vi "Add Panel to SubPanel.vi"(10 "SubPanel Ref":i32, 11 "VI in":refnum<vi>) -> (0 "error out":errorcluster)   [LabVIEW 2015, in "Instrument.lvlib" / "Instrument.lvclass"]
uses:
  Instrument.lvclass
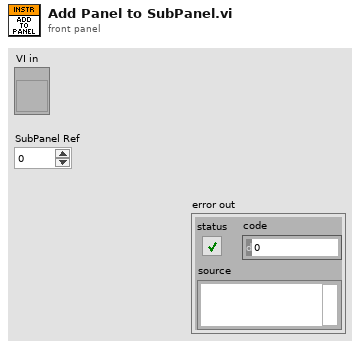
[diagram p1: front panel]
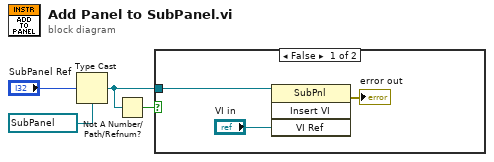
[diagram p0: block diagram]
diagram:
  n1 = Type Cast(type=refnum<vi> refnum ("Sub Panel"), x="SubPanel Ref") -> (*(type *) &x=w1:refnum<vi>)
  n2 = Not A Number/Path/Refnum?(number/path/refnum=w1) -> (NaN/Path/Refnum?=w4:bool)
  n3 = case shown="False" w4 {
    tunnel: w1 -> [w7 _]
    frame False {
      n4 = invoke class="SubPnl" method="Insert VI"(reference=w7, "VI Ref"="VI in") -> (error out=→"error out":errorcluster)  [unwired: 2 in, 3 out]
    }
    frame True {
    }
  }
